vi "Calculate Average Center.vi"(11 "Gantry Fiducials":dbl[](array[numeric])) -> (3 "XYZTheta":dbl[](array[numeric]))   [LabVIEW 2016, in "Component Tray.lvclass"]
uses:
  Component Tray.lvclass
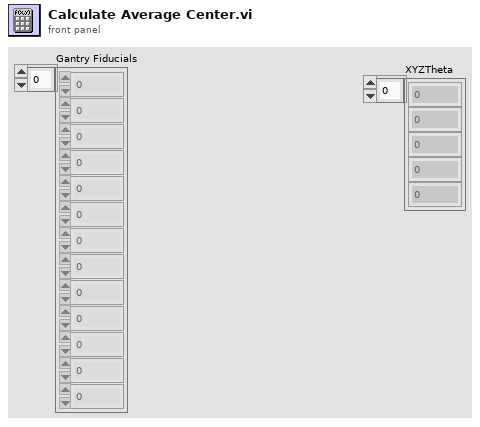
[diagram p1: front panel]
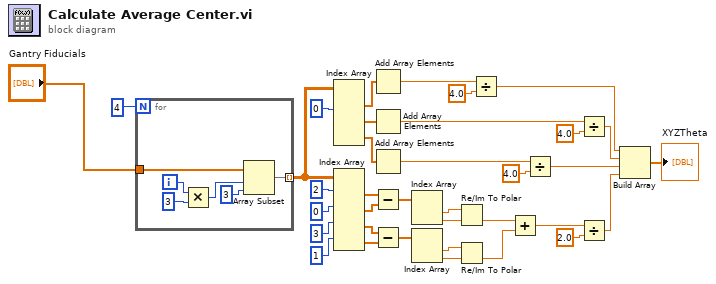
[diagram p0: block diagram]
diagram:
  n1 = for {
    N: 4 -> [_]
    tunnel: "Gantry Fiducials" -> [w38]
    tunnel: [w37] -> w3 mode=indexing
    i -> [w42]
    n2 = Multiply(x=w42, y=3) -> (x*y=w40:i32)
    n3 = Array Subset(array=w38, index=w40, length=3) -> (w37:dbl[])
  }
  n4 = Index Array(array=w3, index (col) #1=0 ("disabled index (col)")) -> (element #1=w35:dbl[], element #2=w34:dbl[], element #3=w1:dbl[])  [unwired: 5 in]
  n5 = Index Array "Index Array"(array=w3, index (row) #1=2 ("index (row)"), index (row) #2=0 ("index (row)"), index (row) #3=3 ("index (row)"), index (row) #4=1 ("index (row)")) -> (element #1=w19:dbl[], element #2=w18:dbl[], element #3=w17:dbl[], element #4=w16:dbl[])  [unwired: 4 in]
  n6 = Add Array Elements(numeric array=w35) -> (sum=w33:dbl)
  n7 = Add Array Elements(numeric array=w34) -> (sum=w32:dbl)
  n8 = Add Array Elements(numeric array=w1) -> (sum=w10:dbl)
  n9 = Subtract(x=w19, y=w18) -> (x-y=w29:dbl[])
  n10 = Subtract(x=w17, y=w16) -> (x-y=w28:dbl[])
  n11 = Index Array(array=w29) -> (element #1=w27:dbl, element #2=w26:dbl)  [unwired: 2 in]
  n12 = Index Array(array=w28) -> (element #1=w25:dbl, element #2=w24:dbl)  [unwired: 2 in]
  n13 = Re/Im To Polar(2:w26, 3:w27) -> (0:w23:dbl)  [unwired: 1 out]
  n14 = Re/Im To Polar(2:w24, 3:w25) -> (0:w22:dbl)  [unwired: 1 out]
  n15 = Divide(x=w33, y=4.0) -> (x/y=w9:dbl)
  n16 = Add(x=w23, y=w22) -> (x+y=w21:dbl)
  n17 = Divide(x=w10, y=4.0) -> (x/y=w7:dbl)
  n18 = Divide(x=w32, y=4.0) -> (x/y=w8:dbl)
  n19 = Divide(x=w21, y=2.0) -> (x/y=w6:dbl)
  n20 = Build Array(w9, w8, w7, w6) -> (→"XYZTheta":dbl[])
